vi "TpSystemEventLevel1.vi"() -> (1 "tracepoint name":string)   [LabVIEW 2017, in "TraceLogger.lvlib"]
uses:
  <vilib>/addons/TraceLogger/TraceLogger.lvlib
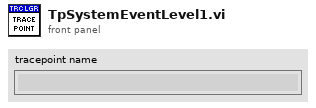
[diagram p1: front panel]
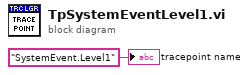
[diagram p0: block diagram]
diagram:
  "tracepoint name" <- "SystemEvent.Level1" ("ProcessName")
